vi "State Manager Test.vi"() -> ()   [LabVIEW 2017]
uses:
  Event.ctl
  State.ctl
panel:
  out "State":T1
  in  "Event":T2=enum."Start Button Pressed"
  in  "Fire Event":bool
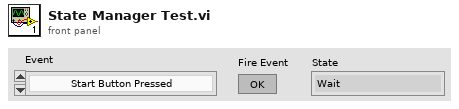
[diagram p1: front panel]
types:
  T1 = typedef "State.ctl" = enum16{"Wait", "Recenter", "Follow Wall", "Zig Zag", "Ramp", "Cross Rough Terrain", "Stagger Stop", "Obstacle Avoidance"}
  T2 = typedef "Event.ctl" = enum16{"None", "Start Obstacle Avoidance", "Start Button Pressed", "Black & Yellow Tape Touched", "Black & Yellow Tape Passed", "Green Tape Crossed", "Red Tape Touched", "Rough Terrain Touched", "Black Tape Crossed", "Tape Edge Too Close", "Wall Too Close", "Rough Terrain Passed", "Ramp Passed", "Stop Button Pressed", "Recentered", "End Zone Wait Timed Out"}
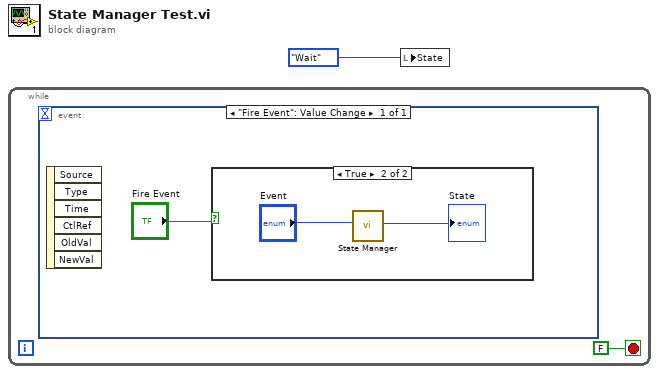
[diagram p0: block diagram]
diagram:
  n1 = while {
    stop <- FALSE stop-if-true
    n2 = event shown="[0] \"Fire Event\": Value Change" {
      selector: _ -> [_]
      dyn-events: _ -> [_]
      timeout: _ -> [_]
      event "Fire Event": Value Change {
        n3 = event-data() -> ()  [unwired: 1 in, 6 out]
        n4 = case shown="True" "Fire Event" {
          frame False {
          }
          frame True {
            n5 = call "State Manager.vi"("Event"="Event") -> ("Next State"=→"State":T1)
          }
        }
      }
    }
  }
  n6 = local write "State"(State."Wait" ("State")) -> ()
